vi "FindInstruments.vi"(8 "error in (no error)":errorcluster, 10 "InstrumentData":T2, 11 "HamaCam in":refnum<class "HamaCam.lvclass">) -> (0 "error out":errorcluster, 3 "HamaCam out":refnum<class "HamaCam.lvclass">)   [LabVIEW 2023, in "HamaCam.lvlib" / "HamaCam.lvclass"]
uses:
  HamaCam.lvclass
  HamaCam.lvclass/HamaCam.ctl
  UIs/InterferometryUI/InterferometryUI/instrumentType.ctl
  Interfaces/InitDeinitInterface/InitDeinitComm Messages/FoundInstruments Msg/FoundInstruments Msg.lvclass
  <vilib>/ActorFramework/Actor/Actor.lvclass
  Applications/National Instruments/LabVIEW 2023 64-bit/vi.lib/ActorFramework/Actor/Actor.lvclass
  Users/alexandrosspiliotis/Documents/LV_DAQ_Project/ConcreteClasses/ConcreteInstrumentClasses/CameraClasses/Hama_LV/HamaCam/HamaCam/HamaCam.lvclass
  Users/alexandrosspiliotis/Documents/LV_DAQ_Project/Interfaces/AbstractInstrumentClasses/Cameras_LV/CameraInterface/CameraInterface.lvclass
  Users/alexandrosspiliotis/Documents/LV_DAQ_Project/Interfaces/InitDeinitInterface/InitDeinit/InitDeinit.lvclass
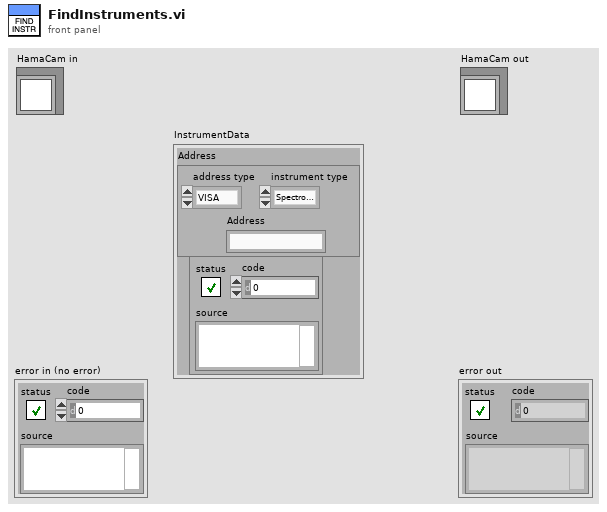
[diagram p1: front panel]
types:
  T1 = typedef "instrumentType.ctl" = enum16{"Spectrometer", "Camera", "Stepper"}
  T2 = cluster{"Instr Error":errorcluster, "Address":cluster{"address type":enum16{"VISA", "Index"}, "Address":string, "instrument type":T1}}
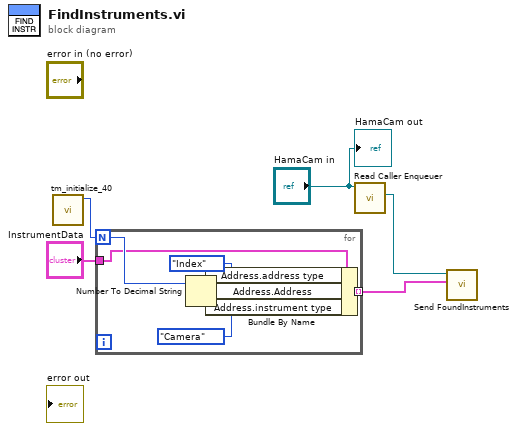
[diagram p0: block diagram]
diagram:
  n1 = call "tm_initialize_40.vi"() -> ("Number Of Cameras"=w5:u32)  [unwired: 8 in, 3 out]
  n2 = for {
    N: w5 -> [w11]
    tunnel: "InstrumentData" -> [w6]
    tunnel: [w7] -> w3 mode=indexing
    n3 = Number To Decimal String(number=w11) -> (decimal integer string=w10:string)  [unwired: 1 in]
    n4 = Bundle By Name(cluster=w6, "Address.address type"=enum16{"VISA", "Index"}."Index" ("address type"), "Address.Address"=w10, "Address.instrument type"=instrumentType."Camera" ("instrument type")) -> (w7:T2)
  }
  n5 = call <vilib>:"Read Caller Enqueuer.vi"("Actor"="HamaCam in") -> ("Caller Enqueuer"=w2:refnum<class "Message Enqueuer.lvclass">)  [unwired: 10 in]
  n6 = call "Send FoundInstruments.vi"("FoundInstruments"=w3, "Message Enqueuer"=w2) -> ()  [unwired: 8 in, 2 out]
  "HamaCam out" <- "HamaCam in"
